vi "View A-Scan.vi"(10 "A-Scan Processed":dbl[](graph), 11 "A-Scan (Raw)":dbl[](graph)) -> ()   [LabVIEW 2014, in "Processing.lvclass"]
uses:
  Processing.lvclass
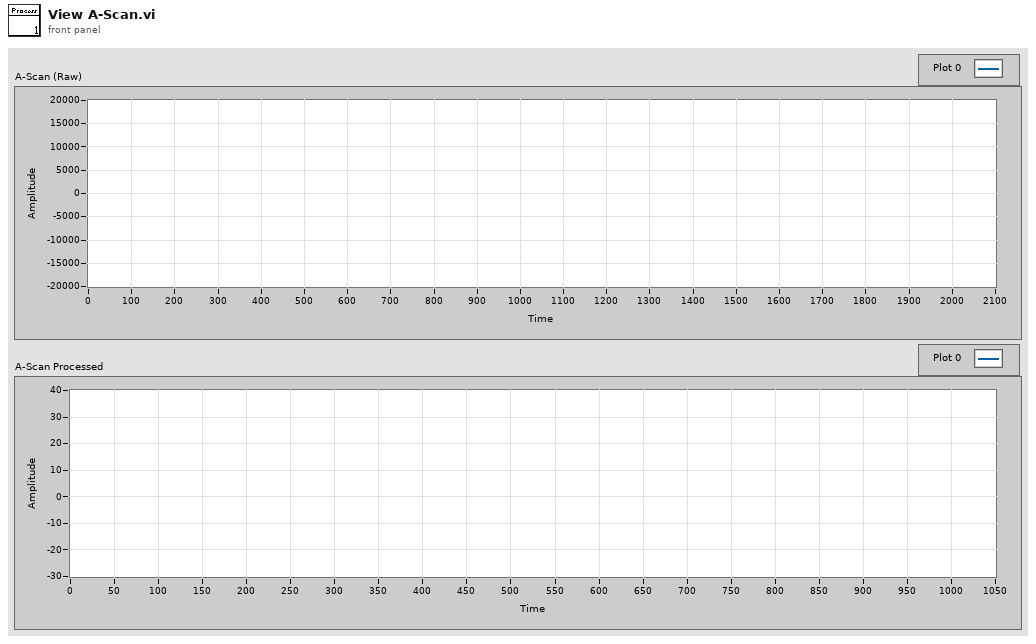
[diagram p1: front panel]
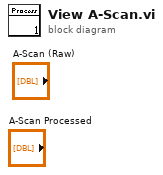
[diagram p0: block diagram]
diagram:
